vi "Temp.vi"() -> ()   [LabVIEW 2018]
panel:
  in  "Table Control 13":string[][](table)=[["", "", "", "1"], ["", "", "", "2"], ["", "", "", "3"], ["", "", "", "4"], ["", "", "", "5"], ["", "", "", "6"], ["", "", "", "7"], ["", "", "", "8"], ["", "", "", "9"], ["", "", "", "10"], ["", "", "", "11"], ["", "", "", "12"], ["", "", "", "13"], ["", "", "", "14"], ["", "", "", "15"], ["", "", "", "16"], ["", "", "", "17"], ["", "", "", "18"], ["", "", "", "19"], ["", "", "", "20"], ["", "", "", "21"], ["", "", "", "22"], ["", "", "", "23"], ["", "", "", "24"]]
  in  "Table Control 12":string[][](table)=[["", "", "", "1"], ["", "", "", "2"], ["", "", "", "3"], ["", "", "", "4"], ["", "", "", "5"], ["", "", "", "6"], ["", "", "", "7"], ["", "", "", "8"], ["", "", "", "9"], ["", "", "", "10"], ["", "", "", "11"], ["", "", "", "12"], ["", "", "", "13"], ["", "", "", "14"], ["", "", "", "15"], ["", "", "", "16"], ["", "", "", "17"], ["", "", "", "18"], ["", "", "", "19"], ["", "", "", "20"], ["", "", "", "21"], ["", "", "", "22"], ["", "", "", "23"], ["", "", "", "24"]]
  in  "Table Control 11":string[][](table)=[["", "", "", "1"], ["", "", "", "2"], ["", "", "", "3"], ["", "", "", "4"], ["", "", "", "5"], ["", "", "", "6"], ["", "", "", "7"], ["", "", "", "8"], ["", "", "", "9"], ["", "", "", "10"], ["", "", "", "11"], ["", "", "", "12"], ["", "", "", "13"], ["", "", "", "14"], ["", "", "", "15"], ["", "", "", "16"], ["", "", "", "17"], ["", "", "", "18"], ["", "", "", "19"], ["", "", "", "20"], ["", "", "", "21"], ["", "", "", "22"], ["", "", "", "23"], ["", "", "", "24"]]
  in  "Table Control":string[][](table)=[["", "", "", "1"], ["", "", "", "2"], ["", "", "", "3"], ["", "", "", "4"], ["", "", "", "5"], ["", "", "", "6"], ["", "", "", "7"], ["", "", "", "8"], ["", "", "", "9"], ["", "", "", "10"], ["", "", "", "11"], ["", "", "", "12"], ["", "", "", "13"], ["", "", "", "14"], ["", "", "", "15"], ["", "", "", "16"], ["", "", "", "17"], ["", "", "", "18"], ["", "", "", "19"], ["", "", "", "20"], ["", "", "", "21"], ["", "", "", "22"], ["", "", "", "23"], ["", "", "", "24"]]
  in  "Boolean 10":bool
  in  "Boolean 9":bool
  in  "Boolean 8":bool
  in  "Boolean 7":bool
  in  "Boolean 6":bool
  in  "Boolean 5":bool
  in  "Boolean 4":bool
  in  "Boolean 3":bool
  in  "Boolean 2":bool
  in  "Boolean":bool
  # "BMS Monitor"
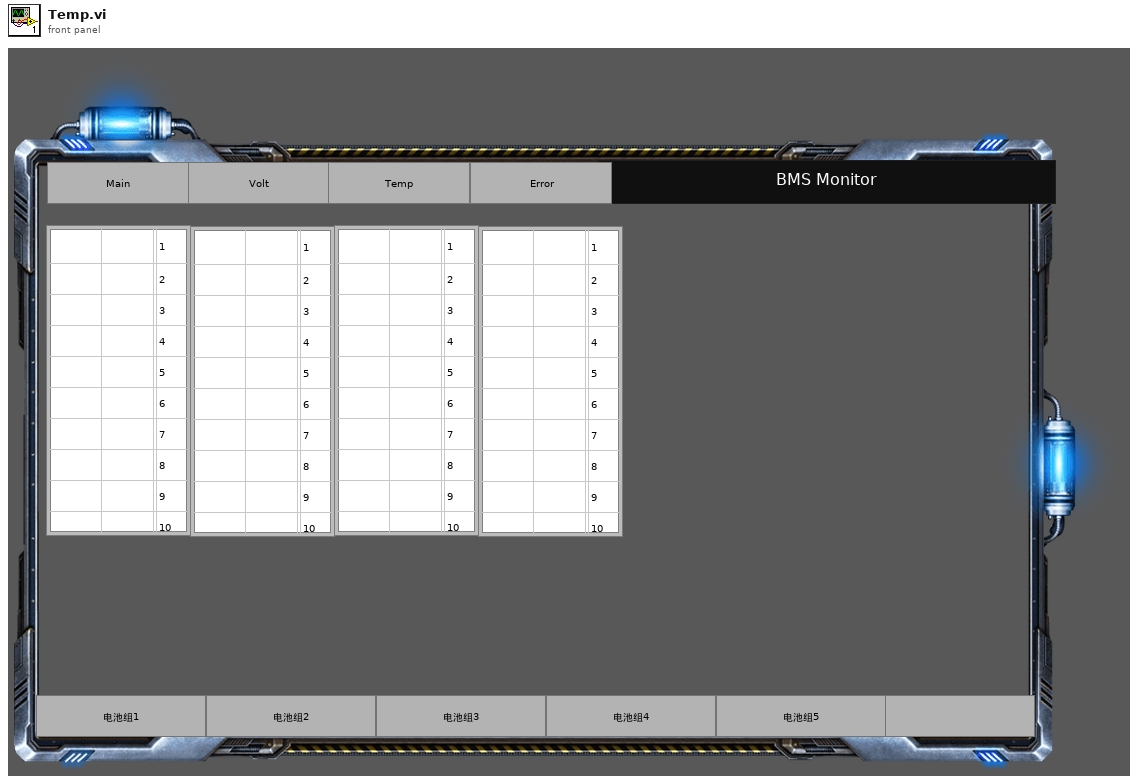
[diagram p1: front panel]
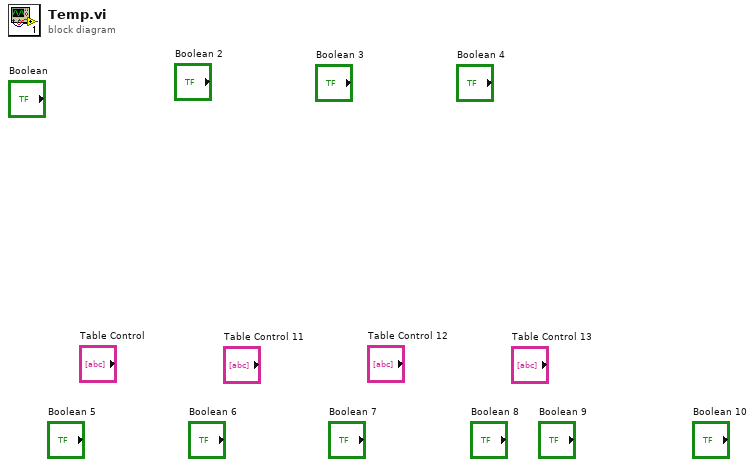
[diagram p0: block diagram]
diagram:
